vi "Router - Latency Bmk - CVT FGV.vi"() -> ()   [LabVIEW 2016]
uses:
  <vilib>/Utility/error.llb/DialogType.ctl
  <vilib>/NI/Current Value Table/Type Defs/File Format.ctl
  <vilib>/NI/Current Value Table/Type Defs/Single Tag.ctl
  <vilib>/NI/Current Value Table/Type Defs/Data Types.ctl
  <vilib>/NI/Current Value Table/Type Defs/Tag Grouping set.ctl
  <vilib>/pximc/Initialize Reader Session (DBL).vi
  <vilib>/pximc/Initialize Writer Session (DBL).vi
  <vilib>/pximc/Connect (DBL).vi
  <vilib>/pximc/Write (DBL).vi
  <vilib>/pximc/Read (DBL).vi
  <vilib>/pximc/nipximc.lvlib
  <vilib>/NI/Current Value Table/Current Value Table.lvlib
panel:
  out "Stopped?":bool
  in  "Node 2 Reader Interface":tag="PXI1Slot2" caption="interface"
  in  "Node 2 Reader Connection ID":u16=4
  in  "Node 2 Writer Interface":tag="PXI1Slot2" caption="interface"
  in  "Node 2 Writer Connection ID":u16=3
  in  "Node 1 Reader Interface":tag="PXI1Slot2" caption="interface"
  in  "Node 1 Reader Connection ID":u16=2
  in  "Stop Button":bool
  in  "Node 1 Writer Interface":tag="PXI1Slot2" caption="interface"
  in  "Buffer Size":u64=250000 caption="buffer size"
  in  "Connection Timeout (s)":dbl=60.0 caption="timeout in seconds (-1)"
  in  "Node 1 Writer Connection ID":u16=1
  # "Node 1"
  # "Node 2"
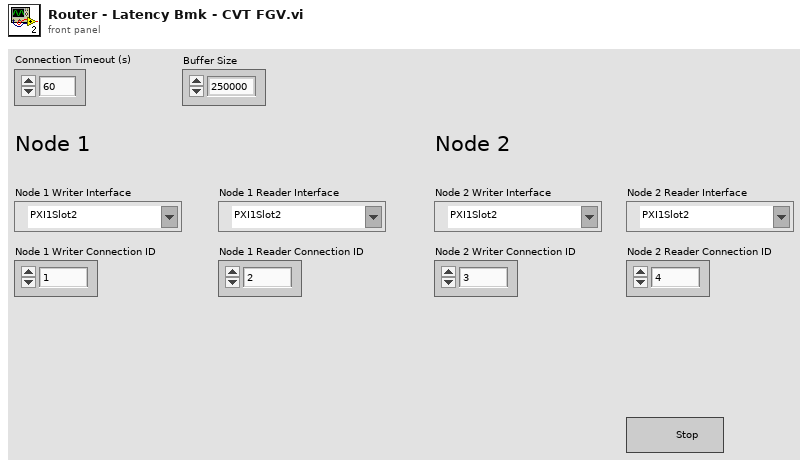
[diagram p1: front panel]
types:
  T1 = typedef "Current Value Table.lvlib/File Format.ctl" = cluster{"Tags":T2[], "Group Listings":T4[]}
  T2 = typedef "Current Value Table.lvlib/Single Tag.ctl" = cluster{"Data Type":T3, "Name":string, "Value":string, "Description":string}
  T3 = typedef "Current Value Table.lvlib/Data Types.ctl" = enum16{"Double", "Single", "I64", "I32", "I16", "I8", "U64", "U32", "U16", "U8", "String", "Boolean", "Array of U8", "Array of U16", "Array of U32", "Array of U64", "Array of I64", "Array of I32", "Array of I16", "Array of I8", "Array of Double", "Array of Single", "Array of Boolean", "Array of String"}
  T4 = typedef "Current Value Table.lvlib/Tag Grouping set.ctl" = cluster{"Group":string, "Tag Names":string[]}
  T5 = typedef "DialogType.ctl" = u16
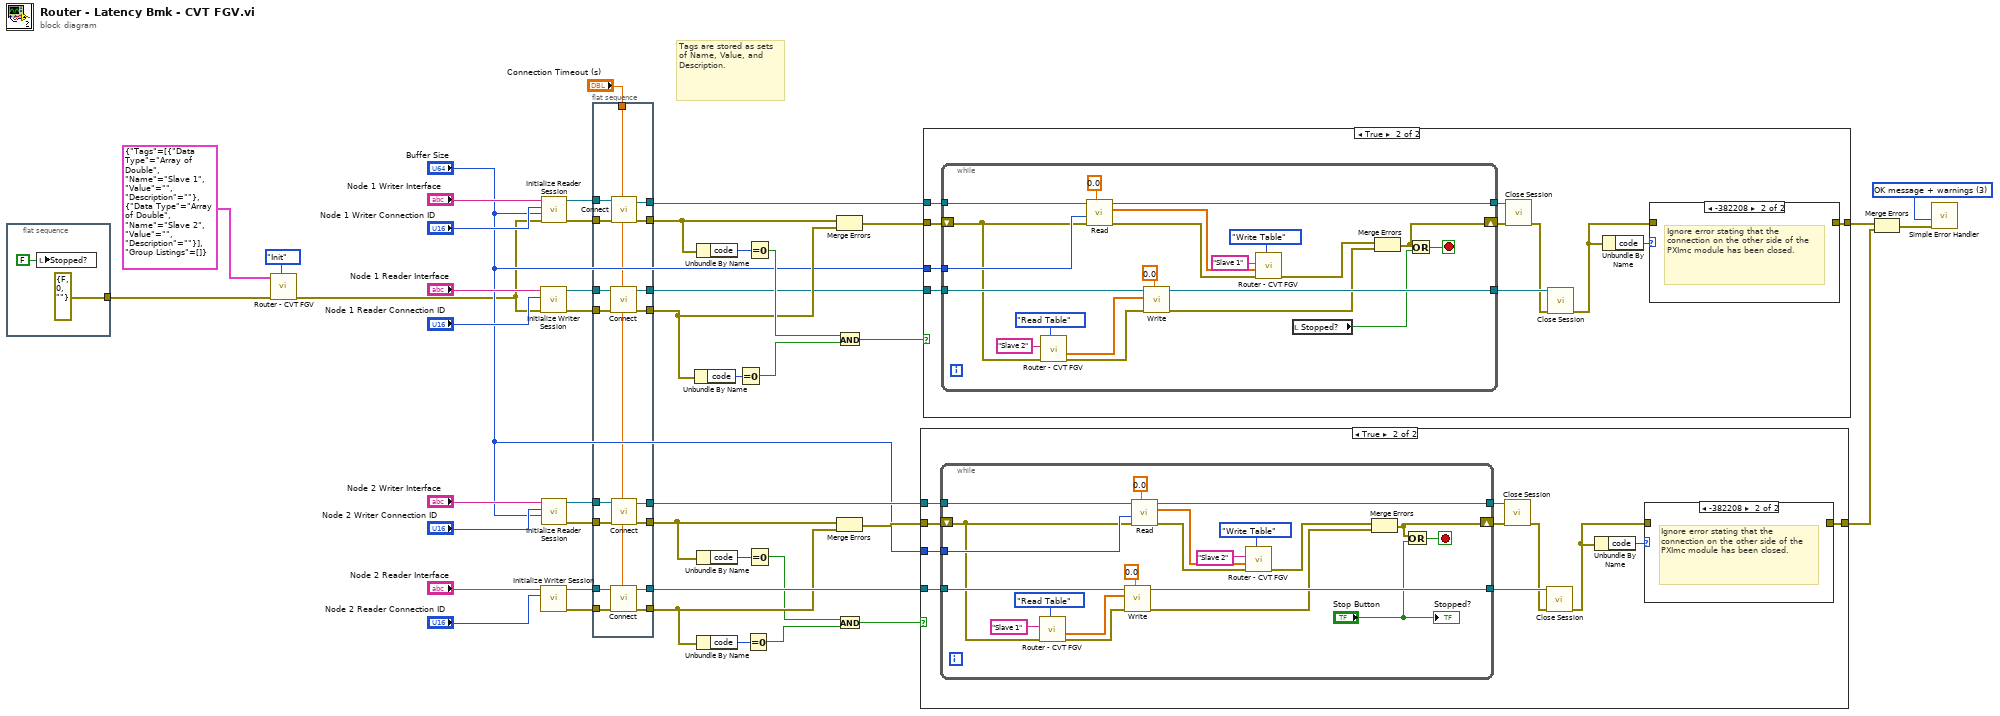
[diagram p0: block diagram]
diagram:
  w40 = T5 3 items=["no dialog", "OK message", "continue or stop message", "OK message + warnings", "continue/stop + warnings"] ("type of dialog (OK msg:1)")
  # "Tags are stored as sets of Name, Value, and Description."
  n1 = flat-sequence {
    tunnel: [errorcluster {"status"=FALSE, "code"=0, "source"=""} ("error constant")] -> w2
    frame #0 {
      n2 = local write "Stopped?"(FALSE ("Stopped?")) -> ()
    }
  }
  n3 = call "Router - CVT FGV.vi"("FGV Command"=enum16{"Init", "Write Table", "Read Table"}."Init", "error in (no error)"=w2, "CVT Tags to Create"=T1 {"Tags"=[{"Data Type"=enum."Array of Double", "Name"="Slave 1", "Value"="", "Description"=""}, {"Data Type"=enum."Array of Double", "Name"="Slave 2", "Value"="", "Description"=""}], "Group Listings"=[]}) -> ("error out"=w1:errorcluster)  [unwired: 7 in, 1 out]
  n4 = call-poly <vilib>:"Initialize Writer Session.vi"("error in (no error)"=w1, "connection id (1)"="Node 1 Reader Connection ID", "interface"="Node 1 Reader Interface") -> ("error out"=w38:errorcluster, "session out"=w37:refnum<k21>)  [unwired: 7 in]
  n5 = call-poly <vilib>:"Initialize Writer Session.vi"("connection id (1)"="Node 2 Reader Connection ID", "interface"="Node 2 Reader Interface") -> ("error out"=w16:errorcluster, "session out"=w17:refnum<k21>)  [unwired: 8 in]
  n6 = call-poly <vilib>:"Initialize Reader Session.vi"("error in (no error)"=w1, "buffer size"="Buffer Size", "writer's connection id (1)"="Node 1 Writer Connection ID", "interface"="Node 1 Writer Interface") -> ("error out"=w44:errorcluster, "session out"=w45:refnum<k21>)  [unwired: 6 in]
  n7 = call-poly <vilib>:"Initialize Reader Session.vi"("buffer size"="Buffer Size", "writer's connection id (1)"="Node 2 Writer Connection ID", "interface"="Node 2 Writer Interface") -> ("error out"=w11:errorcluster, "session out"=w10:refnum<k21>)  [unwired: 7 in]
  n8 = flat-sequence {
    tunnel: w45 -> [w65]
    tunnel: w44 -> [w64]
    tunnel: [w63] -> w43
    tunnel: w38 -> [w62]
    tunnel: w37 -> [w61]
    tunnel: [w60] -> w30
    tunnel: [w59] -> w29
    tunnel: "Connection Timeout (s)" -> [w49]
    tunnel: [w58] -> w27
    tunnel: [w57] -> w26
    tunnel: [w56] -> w25
    tunnel: [w55] -> w24
    tunnel: w17 -> [w54]
    tunnel: w16 -> [w53]
    tunnel: [w52] -> w12
    tunnel: w11 -> [w51]
    tunnel: w10 -> [w50]
    frame #0 {
      n9 = call-poly <vilib>:"Connect.vi"("timeout in seconds (-1)"=w49, "error in (no error)"=w62, "session in"=w61) -> ("error out"=w59:errorcluster, "session out"=w58:refnum<k21>)  [unwired: 7 in]
      n10 = call-poly <vilib>:"Connect.vi"("timeout in seconds (-1)"=w49, "error in (no error)"=w53, "session in"=w54) -> ("error out"=w56:errorcluster, "session out"=w57:refnum<k21>)  [unwired: 7 in]
      n11 = call-poly <vilib>:"Connect.vi"("timeout in seconds (-1)"=w49, "error in (no error)"=w64, "session in"=w65) -> ("error out"=w60:errorcluster, "session out"=w63:refnum<k21>)  [unwired: 7 in]
      n12 = call-poly <vilib>:"Connect.vi"("timeout in seconds (-1)"=w49, "error in (no error)"=w51, "session in"=w50) -> ("error out"=w55:errorcluster, "session out"=w52:refnum<k21>)  [unwired: 7 in]
    }
  }
  n13 = Unbundle By Name(w29) -> ("code"=w35:i32)
  n14 = Unbundle By Name(w30) -> ("code"=w41:i32)
  n15 = Unbundle By Name(w24) -> ("code"=w14:i32)
  n16 = Unbundle By Name(w25) -> ("code"=w19:i32)
  n17 = Equal To 0?(x=w35) -> (x = 0?=w32:bool)
  n18 = Equal To 0?(x=w19) -> (x = 0?=w22:bool)
  n19 = Equal To 0?(x=w41) -> (x = 0?=w33:bool)
  n20 = Equal To 0?(x=w14) -> (x = 0?=w21:bool)
  n21 = Merge Errors(w30, w29) -> (w31:errorcluster)
  n22 = Merge Errors(w24, w25) -> (w23:errorcluster)
  n23 = And(x=w33, y=w32) -> (x .and. y?=w34:bool)
  n24 = And(x=w21, y=w22) -> (x .and. y?=w20:bool)
  n25 = case shown="True" w20 {
    tunnel: w23 -> [w66 w77]
    tunnel: w12 -> [_ w76]
    tunnel: [w66 w74] -> w8
    tunnel: w26 -> [_ w71]
    tunnel: "Buffer Size" -> [_ w67]
    frame False {
      # "The connection was not successful for some reason."
    }
    frame True {
      n26 = while {
        tunnel: w76 -> [w98]
        tunnel: [w97] -> w75
        shift-right: [w92] -> w72
        shift-left: w77 -> [w79]
        tunnel: w71 -> [w96]
        tunnel: [w95] -> w70
        tunnel: w67 -> [w89]
        stop <- w93 stop-if-true
        n27 = call "Router - CVT FGV.vi"("FGV Command"=enum16{"Init", "Write Table", "Read Table"}."Read Table", "error in (no error)"=w79, "Tag Name"="Slave 1") -> ("error out"=w81:errorcluster, "Tag Array Read"=w80:dbl[])  [unwired: 7 in]
        n28 = call-poly <vilib>:"Write.vi"("timeout in seconds (5)"=0.0, "error in (no error)"=w81, "data"=w80, "session in"=w96) -> ("error out"=w94:errorcluster, "session out"=w95:refnum<k21>)  [unwired: 5 in, 1 out]
        n29 = call-poly <vilib>:"Read.vi"("timeout in seconds (5)"=0.0, "error in (no error)"=w79, "number of elements"=w89, "session in"=w98) -> ("error out"=w84:errorcluster, "data"=w83:dbl[], "session out"=w97:refnum<k21>)  [unwired: 5 in]
        n30 = call "Router - CVT FGV.vi"("FGV Command"=enum16{"Init", "Write Table", "Read Table"}."Write Table", "error in (no error)"=w84, "Tag Array Write"=w83, "Tag Name"="Slave 2") -> ("error out"=w82:errorcluster)  [unwired: 6 in, 1 out]
        n31 = Merge Errors(w82, w94) -> (w92:errorcluster)
        n32 = Or(x=w92, y="Stop Button") -> (x .or. y?=w93:bool)
        "Stopped?" <- "Stop Button"
      }
      n33 = call <vilib>:"Close Session.vi"("error in (no error)"=w72, "session in"=w75) -> ("error out"=w69:errorcluster)  [unwired: 9 in]
      n34 = call <vilib>:"Close Session.vi"("error in (no error)"=w69, "session in"=w70) -> ("error out"=w68:errorcluster)  [unwired: 9 in]
      n35 = Unbundle By Name(w68) -> ("code"=w73:i32)
      n36 = case shown="-382208" w73 {
        tunnel: w68 -> [w99 _]
        tunnel: [w99 _] -> w74
        frame 0, Default {
        }
        frame -382208 {
          # "Ignore error stating that the connection on the other side of the PXImc module has been closed."
        }
      }
    }
  }
  n37 = case shown="True" w34 {
    tunnel: w31 -> [w100 w111]
    tunnel: w43 -> [_ w110]
    tunnel: [w100 w108] -> w6
    tunnel: "Buffer Size" -> [_ w105]
    tunnel: w27 -> [_ w104]
    frame False {
      # "The connection was not successful for some reason."
    }
    frame True {
      n38 = while {
        tunnel: w110 -> [w132]
        tunnel: [w131] -> w109
        shift-right: [w125] -> w106
        shift-left: w111 -> [w116]
        tunnel: w105 -> [w130]
        tunnel: w104 -> [w129]
        tunnel: [w128] -> w103
        stop <- w126 stop-if-true
        n39 = call "Router - CVT FGV.vi"("FGV Command"=enum16{"Init", "Write Table", "Read Table"}."Read Table", "error in (no error)"=w116, "Tag Name"="Slave 2") -> ("error out"=w115:errorcluster, "Tag Array Read"=w117:dbl[])  [unwired: 7 in]
        n40 = call-poly <vilib>:"Read.vi"("timeout in seconds (5)"=0.0, "error in (no error)"=w116, "number of elements"=w130, "session in"=w132) -> ("error out"=w114:errorcluster, "data"=w120:dbl[], "session out"=w131:refnum<k21>)  [unwired: 5 in]
        n41 = call-poly <vilib>:"Write.vi"("timeout in seconds (5)"=0.0, "error in (no error)"=w115, "data"=w117, "session in"=w129) -> ("error out"=w127:errorcluster, "session out"=w128:refnum<k21>)  [unwired: 5 in, 1 out]
        n42 = call "Router - CVT FGV.vi"("FGV Command"=enum16{"Init", "Write Table", "Read Table"}."Write Table", "error in (no error)"=w114, "Tag Array Write"=w120, "Tag Name"="Slave 1") -> ("error out"=w113:errorcluster)  [unwired: 6 in, 1 out]
        n43 = local read "Stopped?"() -> (w112:bool)
        n44 = Merge Errors(w113, w127) -> (w125:errorcluster)
        n45 = Or(x=w125, y=w112) -> (x .or. y?=w126:bool)
      }
      n46 = call <vilib>:"Close Session.vi"("error in (no error)"=w106, "session in"=w109) -> ("error out"=w102:errorcluster)  [unwired: 9 in]
      n47 = call <vilib>:"Close Session.vi"("error in (no error)"=w102, "session in"=w103) -> ("error out"=w101:errorcluster)  [unwired: 9 in]
      n48 = Unbundle By Name(w101) -> ("code"=w107:i32)
      n49 = case shown="-382208" w107 {
        tunnel: w101 -> [w133 _]
        tunnel: [w133 _] -> w108
        frame 0, Default {
        }
        frame -382208 {
          # "Ignore error stating that the connection on the other side of the PXImc module has been closed."
        }
      }
    }
  }
  n50 = Merge Errors(w6, w8) -> (w7:errorcluster)
  n51 = call <vilib>:"Simple Error Handler.vi"("type of dialog (OK msg:1)"=w40, "error in (no error)"=w7) -> ()  [unwired: 3 in, 5 out]
